vi "Test Case, Waveform Attributes.vi"() -> ()   [LabVIEW 2010]
uses:
  Generic/Waveform Attribute/Waveform Attribute Cluster.ctl
panel:
  out "processed date and time":timestamp=timestamp(-9593226000 s since 1904-01-01) format="%<%.1X  %x>T "
  out "results":T1[](array[typedef]) {"Value" format="%#.3f"}
  out "input parameters":T1[](array[typedef]) {"Value" format="%#.3f"}
  out "all attributes":T1[](array[typedef]) {"Value" format="%#.3f"}
  in  "error in":errorcluster
  out "error out":errorcluster
  in  "filepath":path=path "C:/5-01-003 Active Electrode Min Max/Waveform 1 -5 mA"
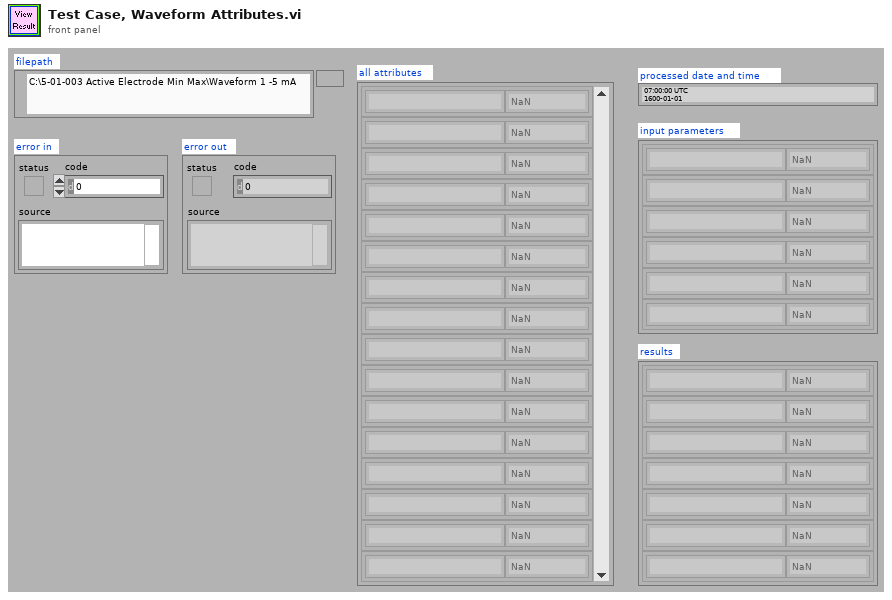
[diagram p1: front panel]
types:
  T1 = typedef "Waveform Attribute Cluster.ctl" = cluster{"Label":string, "Value":dbl}
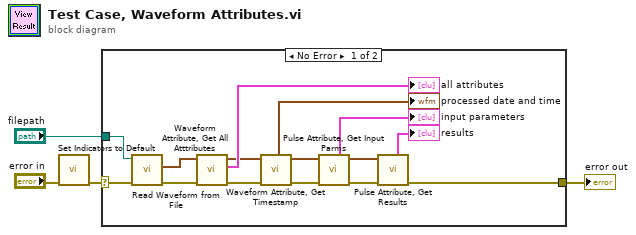
[diagram p0: block diagram]
diagram:
  n1 = call "Set Indicators to Default.vi"("error in"="error in") -> ("error out"=w1:errorcluster)  [unwired: 6 in]
  n2 = case shown="No Error" w1 {
    selector: w1 -> [w19 w20]
    tunnel: "filepath" -> [w18 _]
    tunnel: [w17 w20] -> w3
    frame No Error {
      n3 = call <vilib>:"Read Waveform from File.vi"("error in (no error)"=w19, "file path (dialog if empty)"=w18) -> ("error out"=w11:errorcluster, "first waveform in record"=w10:waveform(dbl))  [unwired: 4 in, 2 out]
      n4 = call "Waveform Attribute, Get All Atttributes.vi"("error in"=w11, "waveform"=w10) -> ("error out"=w7:errorcluster, "all attributes"=→"all attributes":T1[], "waveform dup"=w9:waveform(dbl))  [unwired: 5 in]
      n5 = call "Waveform Attribute, Get Timestamp.vi"("error in"=w7, "waveform"=w9) -> ("error out"=w6:errorcluster, "waveform dup"=w8:waveform(dbl), "Date and Time"=→"processed date and time":timestamp)  [unwired: 4 in, 1 out]
      n6 = call "Pulse Attribute, Get Input Parms.vi"("error in"=w6, "waveform"=w8) -> ("error out"=w16:errorcluster, "waveform dup"=w15:waveform(dbl), "input parameters"=→"input parameters":T1[])  [unwired: 5 in]
      n7 = call "Pulse Attribute, Get Results.vi"("error in"=w16, "waveform"=w15) -> ("error out"=w17:errorcluster, "Results"=→"results":T1[])  [unwired: 5 in, 1 out]
    }
    frame Error {
    }
  }
  "error out" <- w3
